vi "Start_LDA.vi"() -> ()   [LabVIEW 2010]
doc: "The Getting Started Analog Input VI illustrates the basic concepts involved in acquiring analog input data from any data acquisition hardware.\n\nThis VI is explained in detail in the Getting Started with Analog Input section of chapter 1 of the Data Acquisition VI Reference Manual. If you are using SCXI, you should read the Getting Started with SCXI section of chapter 1 first.\n\nAfter you have installed and configured your data acquisition hardware as described in the Installation and Configuration section of chapter 1, you can run this VI to verify your hardware configuration. \n\nYou can pop-up on any front panel object for a description.\n\nIf you are using AMUX-64T boards or SCXI hardware, look at the channels control description for instructions on how to address those external channels; otherwise, you can run the VI with default inputs.\n\nOpen the diagram window to see the data acquisition VI usage."
uses:
  Globals/LDA_meas_global_1.vi
  Globals/Meas_global.vi
  Globals/LDA_meas_global_2.vi
panel:
  in  "Hold for PW to fire (ms)":u32
  out "error out":errorcluster
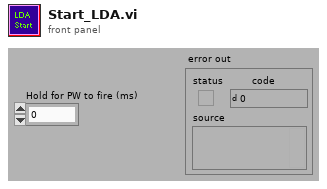
[diagram p1: front panel]
types:
  T1 = typedef "BSA_info_Cluster.ctl" = cluster{"GPIB Address":string, "No of Check Bytes":i32, "Extra Info":string, "COLOUR":u32, "Wavelength (nm)":dbl}
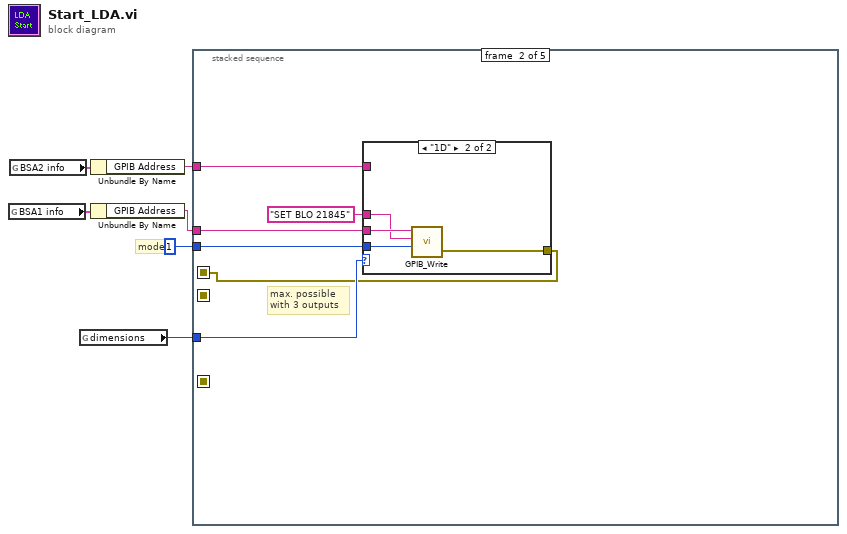
[diagram p0: block diagram]
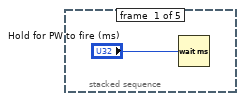
[diagram p2: hidden frame]
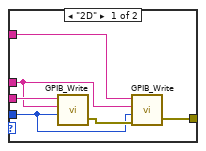
[diagram p3: hidden frame]
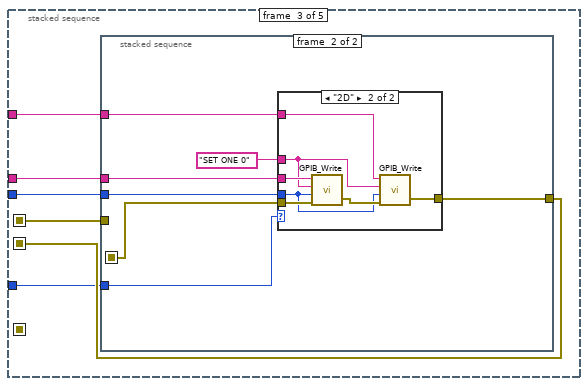
[diagram p4: hidden frame]
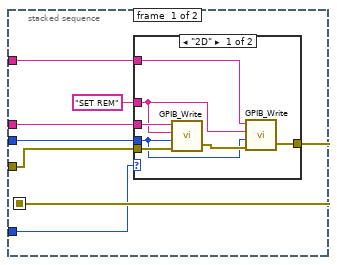
[diagram p5: hidden frame]
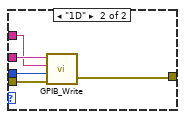
[diagram p6: hidden frame]
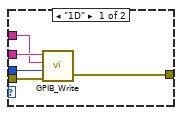
[diagram p7: hidden frame]
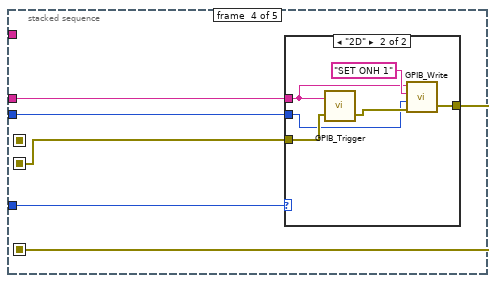
[diagram p8: hidden frame]
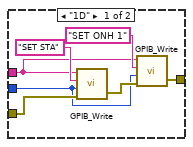
[diagram p9: hidden frame]
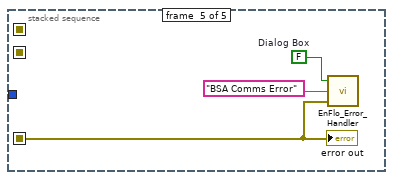
[diagram p10: hidden frame]
diagram:
  # "mode"
  n1 = global read "LDA_meas_global_1.vi" "BSA1 info"() -> (w2:T1)
  n2 = global read "LDA_meas_global_2.vi" "BSA2 info"() -> (w1:T1)
  n3 = global read "Meas_global.vi" "dimensions"() -> (w4:enum16{"1D", "2D"})
  n4 = Unbundle By Name(w1) -> ("GPIB Address"=w3:string)
  n5 = Unbundle By Name(w2) -> ("GPIB Address"=w5:string)
  n6 = stacked-sequence {
    seq-local: [_ w8 _ _ _] -> [_ _ w27 _ _]
    seq-local: [_ _ w26 _ _] -> [_ _ _ w70 _]
    seq-local: [_ _ _ w69 _] -> [_ _ _ _ w86]
    tunnel: w5 -> [_ w13 w28 w68 _]
    tunnel: i16 1 -> [_ w11 w29 w71 _]
    tunnel: w4 -> [_ w10 w25 w72 _]
    tunnel: w3 -> [_ w9 w24 _ _]
    frame #0 {
      n7 = Wait (ms)(milliseconds to wait="Hold for PW to fire (ms)") -> ()  [unwired: 1 out]
    }
    frame #1 {
      # "max. possible with 3 outputs"
      n8 = case shown="\"1D\"" w10 {
        tunnel: w13 -> [w19 w23]
        tunnel: "SET BLO 21845" -> [w17 w21]
        tunnel: w11 -> [w16 w22]
        tunnel: w9 -> [w15 _]
        tunnel: [w14 w20] -> w8
        frame "2D" {
          n9 = call "GPIB_Write.vi"("address string"=w19, "data In"=w17, "mode (0)"=w16) -> ("error out"=w18:errorcluster)  [unwired: 2 in, 1 out]
          n10 = call "GPIB_Write.vi"("address string"=w15, "data In"=w17, "mode (0)"=w16, "error in"=w18) -> ("error out"=w14:errorcluster)  [unwired: 1 in, 1 out]
        }
        frame "1D" {
          n11 = call "GPIB_Write.vi"("address string"=w23, "data In"=w21, "mode (0)"=w22) -> ("error out"=w20:errorcluster)  [unwired: 2 in, 1 out]
        }
      }
    }
    frame #2 {
      n12 = stacked-sequence {
        seq-local: [w31 _] -> [_ w53]
        tunnel: w29 -> [w35 w55]
        tunnel: w28 -> [w36 w54]
        tunnel: w27 -> [w34 _]
        tunnel: [_ w52] -> w26
        tunnel: w25 -> [w30 w51]
        tunnel: w24 -> [w32 w49]
        frame #0 {
          n13 = case shown="\"2D\"" w30 {
            tunnel: w36 -> [w43 w48]
            tunnel: w35 -> [w40 w46]
            tunnel: w34 -> [w42 w47]
            tunnel: "SET REM" -> [w39 w45]
            tunnel: w32 -> [w38 _]
            tunnel: [w37 w44] -> w31
            frame "2D" {
              n14 = call "GPIB_Write.vi"("address string"=w43, "data In"=w39, "mode (0)"=w40, "error in"=w42) -> ("error out"=w41:errorcluster)  [unwired: 1 in, 1 out]
              n15 = call "GPIB_Write.vi"("address string"=w38, "data In"=w39, "mode (0)"=w40, "error in"=w41) -> ("error out"=w37:errorcluster)  [unwired: 1 in, 1 out]
            }
            frame "1D" {
              n16 = call "GPIB_Write.vi"("address string"=w48, "data In"=w45, "mode (0)"=w46, "error in"=w47) -> ("error out"=w44:errorcluster)  [unwired: 1 in, 1 out]
            }
          }
        }
        frame #1 {
          n17 = case shown="\"2D\"" w51 {
            tunnel: w55 -> [w60 w64]
            tunnel: w54 -> [w59 w67]
            tunnel: w53 -> [w58 w66]
            tunnel: [w57 w61] -> w52
            tunnel: "SET ONE 0" -> [w56 w62]
            tunnel: w49 -> [_ w63]
            frame "1D" {
              n18 = call "GPIB_Write.vi"("address string"=w59, "data In"=w56, "mode (0)"=w60, "error in"=w58) -> ("error out"=w57:errorcluster)  [unwired: 1 in, 1 out]
            }
            frame "2D" {
              n19 = call "GPIB_Write.vi"("address string"=w67, "data In"=w62, "mode (0)"=w64, "error in"=w66) -> ("error out"=w65:errorcluster)  [unwired: 1 in, 1 out]
              n20 = call "GPIB_Write.vi"("address string"=w63, "data In"=w62, "mode (0)"=w64, "error in"=w65) -> ("error out"=w61:errorcluster)  [unwired: 1 in, 1 out]
            }
          }
        }
      }
    }
    frame #3 {
      n21 = case shown="\"2D\"" w72 {
        tunnel: w68 -> [w73 w80]
        tunnel: w71 -> [w74 w81]
        tunnel: w70 -> [w79 w83]
        tunnel: [w75 w84] -> w69
        frame "1D" {
          n22 = call "GPIB_Write.vi"("address string"=w73, "data In"="SET STA", "mode (0)"=w74, "error in"=w79) -> ("error out"=w76:errorcluster)  [unwired: 1 in, 1 out]
          n23 = call "GPIB_Write.vi"("address string"=w73, "data In"="SET ONH 1", "mode (0)"=w74, "error in"=w76) -> ("error out"=w75:errorcluster)  [unwired: 1 in, 1 out]
        }
        frame "2D" {
          n24 = call "GPIB_Trigger.vi"("error in"=w83, "address string"=w80) -> ("error out"=w82:errorcluster)  [unwired: 1 out]
          n25 = call "GPIB_Write.vi"("address string"=w80, "data In"="SET ONH 1", "mode (0)"=w81, "error in"=w82) -> ("error out"=w84:errorcluster)  [unwired: 1 in, 1 out]
        }
      }
    }
    frame #4 {
      w88 = FALSE  # Dialog Box
      n26 = call "EnFlo_Error_Handler.vi"("error in (no error)"=w86, "Error Type"="BSA Comms Error", "Dialog Box (T)"=w88) -> ()  [unwired: 3 out]
      "error out" <- w86
    }
  }
